vi "BlackBox_filtered.vi"() -> ()   [LabVIEW 2019]
uses:
  <vilib>/Analysis/Matrix/Datatypes/RealMatrix.ctl
  <vilib>/userDefined/High Color/IMAQdx.ctl
  <vilib>/Platform/TimedLoop/XDataNode/timing_clust.ctl
  <vilib>/Platform/TimedLoop/XDataNode/nitl_modes.ctl
  <vilib>/Platform/TimedLoop/XDataNode/wakeup.ctl
  <vilib>/myRIO/Instrument Drivers/Onboard IO/AO/typedefs/AO Reference.ctl
  <vilib>/myRIO/Common/Instrument Driver Framework/Utilities/typedefs/myRIO Generic Hardware Reference.ctl
  <vilib>/myRIO/Common/Instrument Driver Framework/Utilities/typedefs/Hardware Version Enum.ctl
  <vilib>/myRIO/Common/Instrument Driver Framework/Utilities/typedefs/myRIO v1.0 Reference.ctl
  <vilib>/myRIO/Common/Instrument Driver Framework/Utilities/typedefs/Generic FPGA Reference.ctl
  <vilib>/myRIO/Common/Instrument Driver Framework/myRIO v1.0/AO/typedefs/AO Channels List.ctl
  <vilib>/myRIO/Common/Instrument Driver Framework/myRIO v1.0/AO/typedefs/AO Channels Enum.ctl
  <vilib>/myRIO/Common/Instrument Driver Framework/Utilities/typedefs/Analog Scaling Constants List.ctl
  <vilib>/myRIO/Common/Instrument Driver Framework/Utilities/typedefs/Analog Scaling Constants.ctl
  <vilib>/userDefined/High Color/nirio_resource_hc.ctl
  <vilib>/myRIO/Common/Instrument Driver Framework/myRIO v1.0/Encoder/typedefs/Encoder Signal Mode.ctl
  <vilib>/myRIO/Instrument Drivers/Onboard IO/Encoder/typedefs/Encoder Reference.ctl
  <vilib>/myRIO/Common/Instrument Driver Framework/myRIO v1.0/Encoder/typedefs/Encoder Channels Enum.ctl
  <vilib>/myRIO/Common/Instrument Driver Framework/myRIO v1.0/Encoder/typedefs/Encoder Configuration v1.0.ctl
  <vilib>/myRIO/Common/Instrument Driver Framework/Utilities/vis/Is FPGA Ref Available.vi
  <vilib>/myRIO/Common/Instrument Driver Framework/myRIO v1.0/AO/vis/myRIO v1.1 Open AO.vi
  <vilib>/myRIO/Instrument Drivers/Onboard IO/AO/vis/Write.vi
  <vilib>/myRIO/Common/Instrument Driver Framework/myRIO v1.0/Encoder/vis/myRIO v1.1 Open Encoder.vi
  <vilib>/myRIO/Instrument Drivers/Onboard IO/Encoder/vis/Read.vi
  <vilib>/myRIO/Common/Instrument Driver Framework/Utilities/vis/Validate Channels.vi
  <vilib>/myRIO/Common/Instrument Driver Framework/myRIO v1.0/AO/vis/myRIO v1.0 Reserve AO.vi
  <vilib>/myRIO/Common/Instrument Driver Framework/myRIO v1.0/Encoder/vis/myRIO v1.0 Reserve Encoder.vi
  <vilib>/Analysis/baseanly.llb/A x B.vi
  <vilib>/Analysis/baseanly.llb/A x Vector.vi
  <vilib>/myRIO/Common/Instrument Driver Framework/myRIO v1.0/AO/vis/myRIO v1.0 Build MUX Configuration AO.vi
  <vilib>/myRIO/Common/Instrument Driver Framework/myRIO v1.0/Resource Manager/vis/myRIO v1.0 Reserve Channel List.vi
  <vilib>/myRIO/Common/Instrument Driver Framework/myRIO v1.0/Encoder/vis/myRIO v1.0 Build MUX Configuration Encoder.vi
  <vilib>/myRIO/Common/Instrument Driver Framework/myRIO v1.0/Resource Manager/vis/myRIO v1.0 Reserve Channel.vi
  <vilib>/myRIO/Common/Instrument Driver Framework/myRIO v1.0/Resource Manager/vis/myRIO v1.0 Unreserve Channel.vi
  <vilib>/myRIO/Common/Instrument Driver Framework/myRIO v1.0/Resource Manager/vis/myRIO v1.0 Create Configuration List.vi
  <vilib>/myRIO/Common/Instrument Driver Framework/myRIO v1.0/Resource Manager/vis/myRIO v1.0 Build Mutex Name.vi
  <vilib>/Utility/VariantDataType/GetNumericInfo.vi
  <vilib>/Utility/error.llb/Error Cluster From Error Code.vi
  <vilib>/myRIO/Common/Instrument Driver Framework/myRIO v1.0/myRIO v1.1 Open.vi
  <vilib>/myRIO/Common/Instrument Driver Framework/myRIO v1.0/AO/vis/myRIO v1.0 Get Scaling Constants AO.vi
  <vilib>/myRIO/Common/Instrument Driver Framework/Utilities/vis/IO Manager.vi
  <vilib>/myRIO/Common/Instrument Driver Framework/Utilities/vis/Configuration Manager.vi
  <vilib>/myRIO/Common/Instrument Driver Framework/myRIO v1.0/myRIO v1.0 Close.vi
  <vilib>/myRIO/Common/Instrument Driver Framework/myRIO v1.0/AO/vis/myRIO v1.0 Write AO.vi
  <vilib>/Utility/file.llb/Write Delimited Spreadsheet (DBL).vi
  <vilib>/myRIO/Common/Instrument Driver Framework/myRIO v1.0/Resource Manager/vis/myRIO v1.0 Configure IO.vi
  <vilib>/myRIO/Common/Instrument Driver Framework/myRIO v1.0/Encoder/vis/myRIO v1.0 Configure Encoder.vi
  <vilib>/myRIO/Common/Instrument Driver Framework/myRIO v1.0/Encoder/vis/myRIO v1.0 Read Encoder.vi
  <vilib>/platform/TimedLoop/XDataNode/XDataNode.xnode
  <vilib>/myRIO/Express VI/Onboard IO/AO/AO Express VI.xnode
  <vilib>/myRIO/Instrument Drivers/Onboard IO/AO/vis/myRIO AO Open.xnode
  <vilib>/myRIO/Express VI/Onboard IO/Encoder/Encoder Express VI.xnode
  <vilib>/myRIO/Instrument Drivers/Onboard IO/Encoder/vis/myRIO Encoder Open.xnode
  <vilib>/myRIO/Common/Instrument Driver Framework/myRIO v1.0/Encoder/typedefs/Encoder Count Direction Enum.ctl
  <vilib>/Platform/TimedLoop/XDataNode/XDNodeRunTimeDep.lvlib
  <vilib>/myRIO/Instrument Drivers/Onboard IO/AO/AO.lvlib
  <vilib>/vision/driver/NI_Vision_Acquisition_Software.lvlib
  <vilib>/myRIO/Instrument Drivers/Onboard IO/Encoder/Encoder.lvlib
  <vilib>/vision/NI_Vision_Development_Module.lvlib
  <vilib>/Analysis/Matrix/NI_Matrix.lvlib
panel:
  out "deltaT":u32
  out "scaled_obs_y":dbl[](array[numeric])
  out "scaled_obs_x":dbl[](array[numeric])
  out "done":bool
  out "target_y":dbl
  out "target_x":dbl
  in  "start_test":bool
  out "observation":dbl[](array[numeric])
  out "scaled_obs":dbl[](array[numeric])
  in  "record_name":string
  out "record":T1
  out "step_recorded":dbl
  in  "stop_recording":bool
  in  "start_recording":bool
  out "recording":bool
  out "record_t":dbl[](array[numeric])
  out "target_a_y":dbl(knob) scale=-45.0..45.0
  out "target_a_x":dbl(knob) scale=-45.0..45.0
  out "y_angle":dbl(knob) scale=-45.0..45.0
  out "x_angle":dbl(knob) scale=-45.0..45.0
  out "y_error":dbl
  out "x_error":dbl
  out "y":dbl
  out "x":dbl
  out "camera":T2(plugin-control)
  in  "threshold":cluster{"Lower value":sgl, "Upper value":sgl}={"Lower value"=60.0, "Upper value"=255.0} {"Upper value" format="%.2f"; "Lower value" format="%.2f"}
  out "threshold":T2(plugin-control)
  out "x-y":u32
  out "y_input":dbl
  out "y_angle_error":dbl
  out "x_angle_error":dbl
  in  "stop":bool
  out "x_input":dbl
  in  "reset":bool
  in  "dt":dbl=20.0
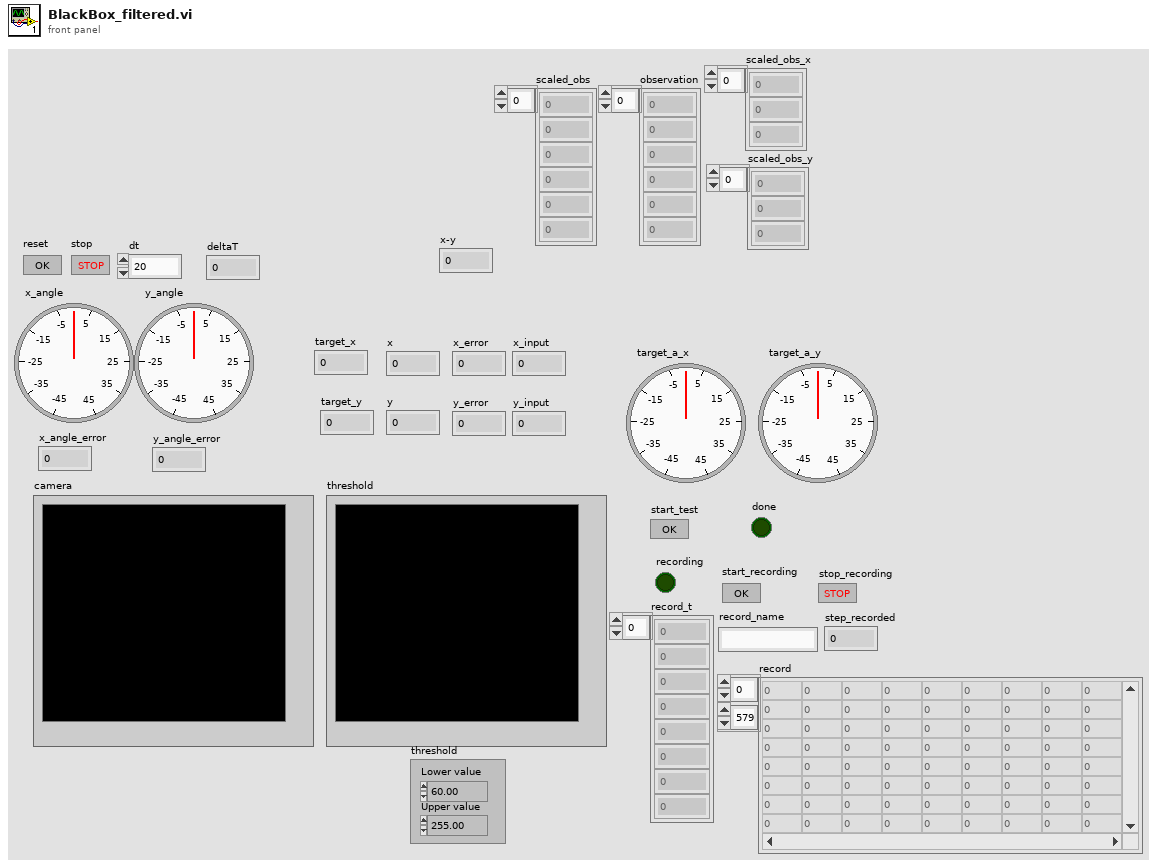
[diagram p1: front panel]
types:
  T1 = typedef "NI_Matrix.lvlib/RealMatrix.ctl" = dbl[][]
  T2 = typedef "IMAQ Image.ctl" = refnum<image>
  T3 = typedef "IMAQdx.ctl" = refnum<k21>
  T4 = typedef "XDNodeRunTimeDep.lvlib/timing_clust.ctl" = cluster{"Expected End [f-1]":u64, "Actual End [f-1]":u64, "Finished Late? [f-1]":bool, "Expected End [i-1]":u64, "Actual End [i-1]":u64, "Finished Late? [i-1]":bool, "Expected Start [i]":u64, "Actual Start [i]":u64, "Expected Start [f]":u64, "Actual Start [f]":u64, "Source Name":string, "Structure Name":string, "Period":i64, "Deadline":i64, "Offset":i64, "Start":i64, "Priority":i32, "Timeout":i32, "Mode":T5, "Wakeup Reason":T6, "Error":errorcluster, "Source Type":string, "Secondary Source Type":string, "Global End Time":u64, "Global Start Time":u64, "Frame Duration":u64, "Iteration Duration":u64, "Assigned CPU":i32, "I/O Scan Engine Mode":u32}
  T5 = typedef "XDNodeRunTimeDep.lvlib/nitl_modes.ctl" = enum32{"No Change", "Process missed periods, maintain original phase", "Discard missed periods, maintain original phase", "Process missed periods, ignore original phase", "Discard missed periods, ignore original phase"}
  T6 = typedef "XDNodeRunTimeDep.lvlib/wakeup.ctl" = enum32{"Normal", "Aborted", "Asynchronous wakeup", "Timing source error", "Timed loop error", "Timeout"}
  T7 = typedef "Encoder.lvlib/Encoder Reference.ctl" = cluster{"myRIO Reference":T8, "Encoder Channels Enum":T12}
  T8 = typedef "myRIO Generic Hardware Reference.ctl" = cluster{"myRIO Model":T9, "myRIO Hardware Reference":T10}
  T9 = typedef "Hardware Version Enum.ctl" = enum16{"Unknown", "myRIO-1900", "myRIO-1950", "roboRIO", "NI ELVIS RIO CM", "ELVIS III"}
  T10 = typedef "myRIO v1.0 Reference.ctl" = cluster{"Generic FPGA Reference":T11, "Allow multiple opens":bool}
  T11 = typedef "Generic FPGA Reference.ctl" = refnum<k20>
  T12 = typedef "Encoder Channels Enum.ctl" = enum16{"Not Connected", "C/ENC0", "C/ENC1", "A/ENC", "A/ENC0", "A/ENC1", "A/ENC2", "A/ENC3", "A/ENC4", "A/ENC5", "A/ENC6", "A/ENC7", "A/ENC8", "A/ENC9", "B/ENC", "B/ENC0", "B/ENC1", "B/ENC2", "B/ENC3", "B/ENC4", "B/ENC5", "B/ENC6", "B/ENC7", "B/ENC8", "B/ENC9", "DIO/ENC0", "DIO/ENC1", "DIO/ENC2", "DIO/ENC3", "DIO/ENC4"}
  T13 = typedef "Encoder Signal Mode.ctl" = enum16{"Quadrature phase signal", "Step and direction signal"}
  T14 = typedef "nirio_resource_hc.ctl" = tag
  T15 = typedef "AO.lvlib/AO Reference.ctl" = cluster{"myRIO Reference":T8, "AO Channel List":T16, "AO Scaling Constant List":T18}
  T16 = typedef "AO Channels List.ctl" = T17[]
  T17 = typedef "AO Channels Enum.ctl" = enum16{"Not Connected", "AudioOut/Left", "AudioOut/Right", "C/AO0", "C/AO1", "A/AO0", "A/AO1", "B/AO0", "B/AO1"}
  T18 = typedef "Analog Scaling Constants List.ctl" = T19[]
  T19 = typedef "Analog Scaling Constants.ctl" = cluster{"LSB Weight (Volts)":dbl, "Offset (Volts)":dbl, "Signed?":bool}
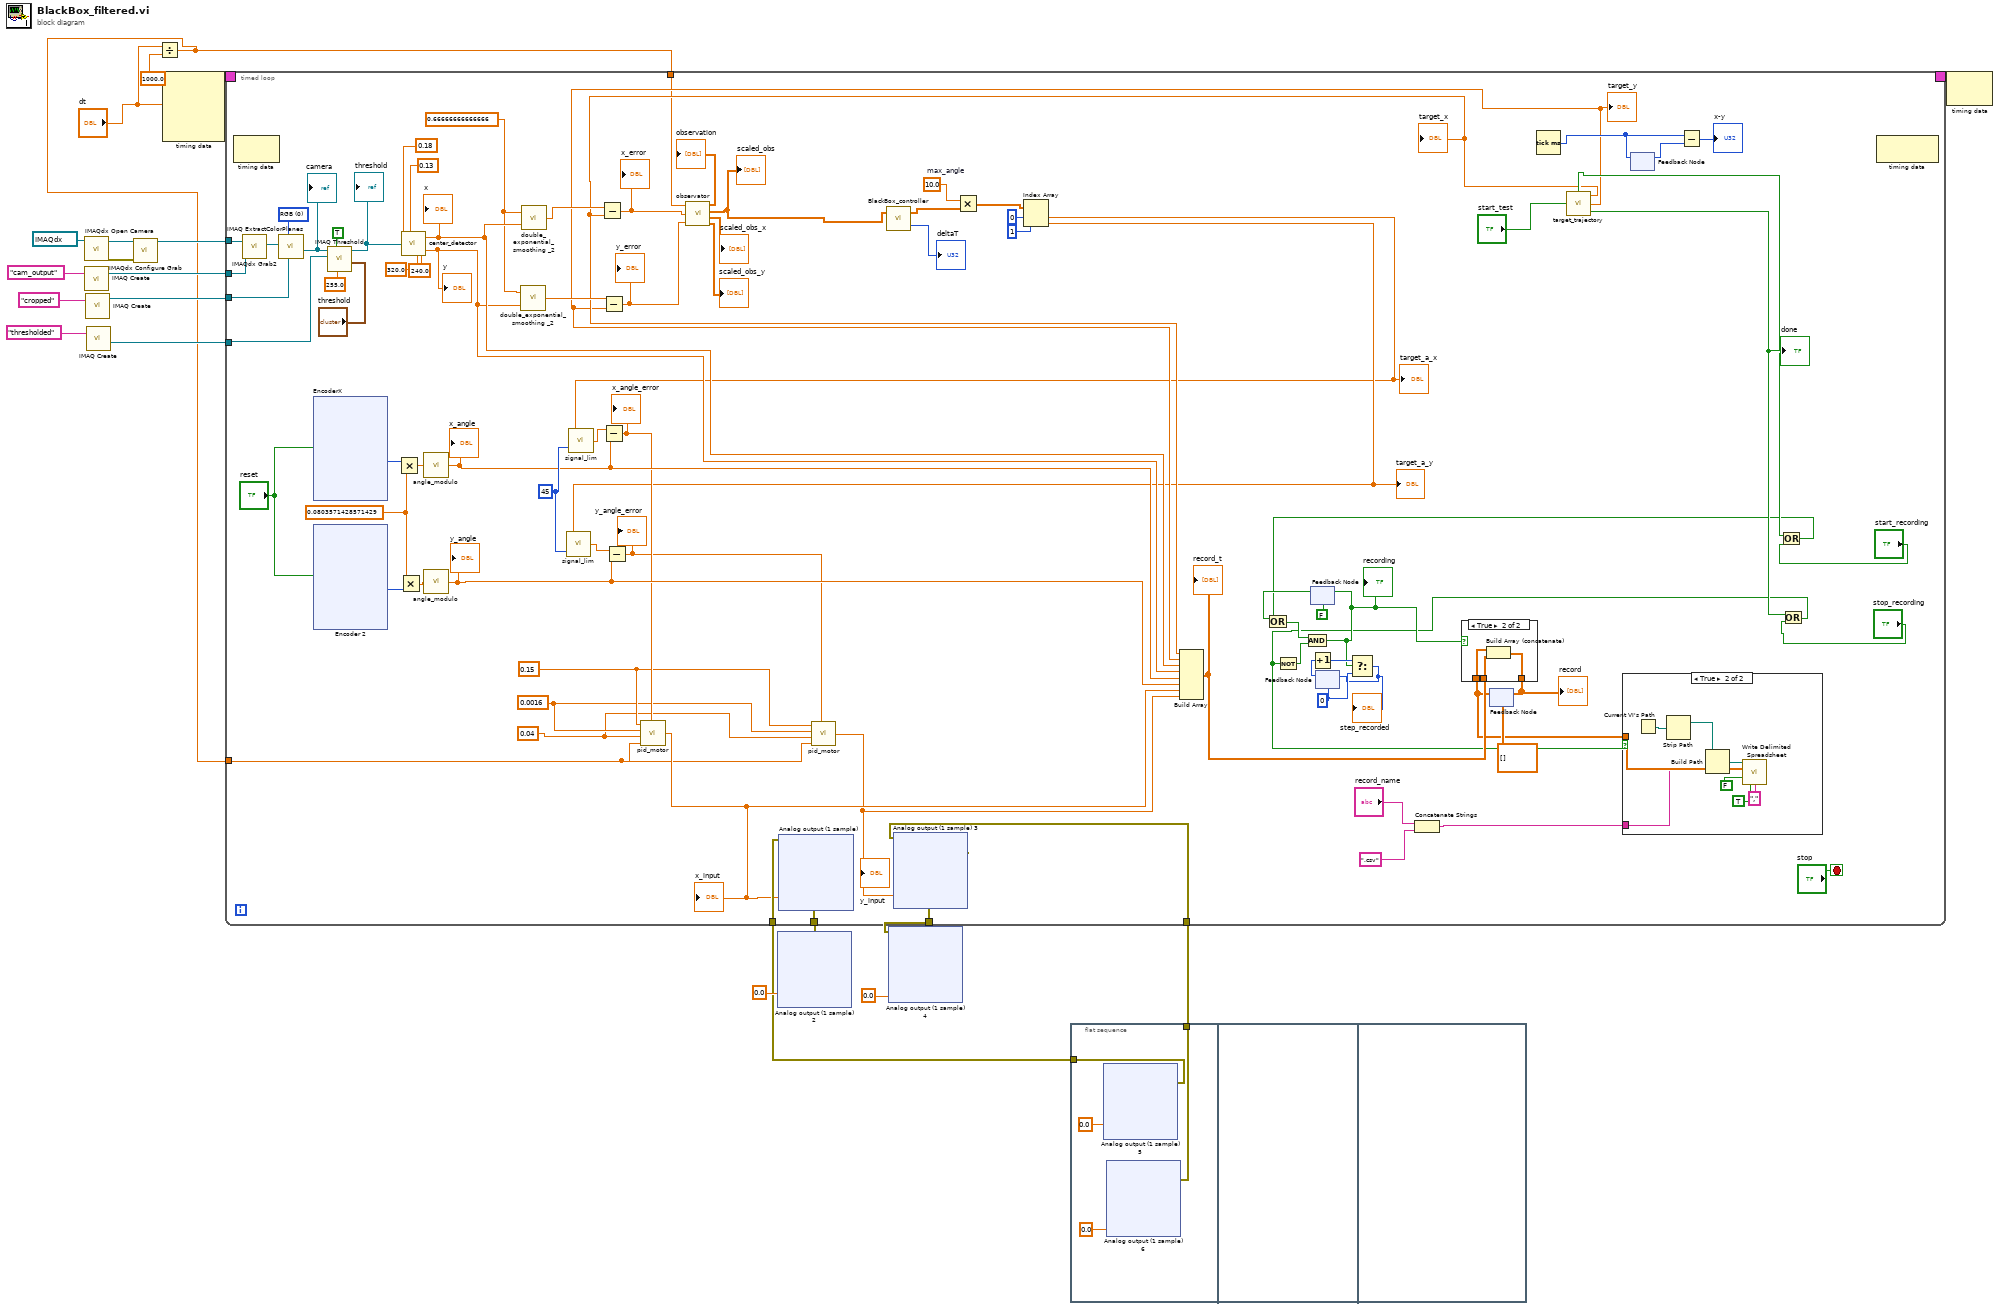
[diagram p0: block diagram]
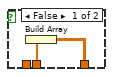
[diagram p3: hidden frame]
diagram:
  n1 = call <vilib>:"IMAQdx Open Camera.vi"("Session In"=T3 "cam2") -> ("error out"=w13:errorcluster, "Session Out"=w14:T3)  [unwired: 9 in]
  n2 = call "IMAQ Create"("Image Name"="cam_output") -> ("New Image"=w15:T2)  [unwired: 4 in, 1 out]
  n3 = call "IMAQ Create"("Image Name"="cropped") -> ("New Image"=w6:T2)  [unwired: 4 in, 1 out]
  n4 = call "IMAQ Create"("Image Name"="thresholded") -> ("New Image"=w4:T2)  [unwired: 4 in, 1 out]
  n5 = call <vilib>:"IMAQdx Configure Grab.vi"("error in"=w13, "Session In"=w14) -> ("Session Out"=w16:T3)  [unwired: 8 in, 1 out]
  n6 = Divide(x="dt", y=1000.0) -> (x/y=w1:dbl)
  n7 = node-c288("dt") -> (w21:T4)  [unwired: 3 in]
  n8 = timed-loop {
    timing: w21 -> [_]
    timing-out: [_] -> w20
    tunnel: w16 -> [w108]
    tunnel: w15 -> [w107]
    tunnel: w1 -> [w49]
    tunnel: [w96] -> w11
    tunnel: [w92] -> w10
    tunnel: w9 -> [w91]
    tunnel: w8 -> [w90]
    tunnel: w6 -> [w65]
    tunnel: w4 -> [w59]
    tunnel: w1 -> [w37]
    stop <- "stop" stop-if-true
    w23 = 10.0  # max_angle
    w54 = 0.66666666666666
    w46 = 0.04 ("ki")
    w47 = 0.0016 ("kd")
    w48 = 0.15 ("kp")
    w68 = u16 0 items=["RGB", "HSL", "HSV", "HSI"] ("Color Mode")
    w78 = 0
    w97 = 45
    w105 = 0.0803571428571429
    n9 = node-c288() -> ()  [unwired: 1 in, 1 out]
    n10 = call <vilib>:"IMAQdx Grab2.vi"("Image In"=w107, "Session In"=w108) -> ("Image Out"=w67:T2)  [unwired: 6 in, 3 out]
    n11 = call "IMAQ ExtractColorPlanes"("Blue or Luma or Val or Inten Plane"=w65, "Color Mode"=w68, "Image Src"=w67) -> ("Blue or Luma or Val or Inten Plane out"=w66:T2)  [unwired: 5 in, 3 out]
    "camera" <- w66
    n12 = xnode "EncoderX"("Reset Counter"="reset") -> ("Counter Value"=w106:i32)  [unwired: 1 in, 3 out]
    n13 = xnode "Encoder 2"("Reset Counter"="reset") -> ("Counter Value"=w104:i32)  [unwired: 1 in, 3 out]
    n14 = call "IMAQ Threshold"("Replace Value"=sgl 255.0, "Keep/Replace Value (Replace)"=TRUE, "Range"="threshold", "Image Dst"=w59, "Image Src"=w66) -> ("Image Dst Out"=w62:T2)  [unwired: 5 in, 1 out]
    "threshold" <- w62
    n15 = Multiply(x=w106, y=w105) -> (x*y=w101:dbl)
    n16 = Multiply(x=w105, y=w104) -> (x*y=w100:dbl)
    n17 = call "center_detector.vi"("px_x"=320.0, "px_y"=240.0, "Image"=w62, "m_x"=0.18, "m_y"=0.13) -> ("x"=w57:dbl, "y"=w55:dbl)
    "x" <- w57
    "y" <- w55
    n18 = call "angle_modulo.vi"("alpha"=w101) -> ("alpha_prime"=w86:dbl)
    "x_angle" <- w86
    n19 = call "angle_modulo.vi"("alpha"=w100) -> ("alpha_prime"=w85:dbl)
    "y_angle" <- w85
    n20 = call "double_exponential_smoothing _2.vi"("x"=w55, "alpha"=w54) -> ("dema"=w56:dbl)
    n21 = call "double_exponential_smoothing _2.vi"("x"=w57, "alpha"=w54) -> ("dema"=w58:dbl)
    n22 = feedback #1(FALSE) -> (w84:bool)
    n23 = feedback #2(w78) -> (w80:i32)
    n24 = Increment(x=w80) -> (x+1=w79:i32)
    n25 = Concatenate Strings("record_name", ".csv") -> (w69:string)
    n26 = feedback #3(T1 [] ("Real Matrix")) -> (w72:T1)
    n27 = Tick Count (ms)() -> (millisecond timer value=w95:u32)
    n28 = call "target_trajectory.vi"("start_test"="start_test") -> ("start"=w42:bool, "target_x"=w39:dbl, "target_y"=w38:dbl, "done"=w43:bool)
    "target_x" <- w39
    "target_y" <- w38
    "done" <- w43
    n29 = Subtract(x=w58, y=w39) -> (x-y=w36:dbl)
    "x_error" <- w36
    n30 = Subtract(x=w56, y=w38) -> (x-y=w35:dbl)
    "y_error" <- w35
    n31 = call "observator.vi"("d_t"=w37, "e_x"=w36, "e_y"=w35) -> ("observation"=→"observation":dbl[], "scaled_obs"=w30:dbl[], "scaled_obs_x"=→"scaled_obs_x":dbl[], "scaled_obs_y"=→"scaled_obs_y":dbl[])
    "scaled_obs" <- w30
    n32 = call "BlackBox_controller.vi"("Normalized observation"=w30) -> ("deltaT"=→"deltaT":u32, "output"=w24:dbl[])  [unwired: 1 in]
    n33 = Multiply(x=w23, y=w24) -> (x*y=w22:dbl[])
    n34 = Index Array(array=w22, index #1=0 ("index"), index #2=1 ("index")) -> (element #1=w25:dbl, element #2=w26:dbl)
    "target_a_x" <- w25
    "target_a_y" <- w26
    n35 = call "signal_lim.vi"("lim"=w97, "x"=w26) -> ("y"=w98:dbl)
    n36 = call "signal_lim.vi"("lim"=w97, "x"=w25) -> ("y"=w99:dbl)
    n37 = Subtract(x=w99, y=w86) -> (x-y=w53:dbl)
    "x_angle_error" <- w53
    n38 = Subtract(x=w98, y=w85) -> (x-y=w51:dbl)
    "y_angle_error" <- w51
    n39 = call "pid_motor.vi"("kp"=w48, "kd"=w47, "ki"=w46, "dt"=w49, "err"=w53) -> ("u"=w52:dbl)
    "x_input" <- w52
    n40 = xnode "Analog output (1 sample)"("C/AO0 (AO0)"=w52, "error in (no error)"=w91) -> ("error out"=w96:errorcluster)
    n41 = call "pid_motor.vi"("kp"=w48, "kd"=w47, "ki"=w46, "dt"=w49, "err"=w51) -> ("u"=w50:dbl)
    "y_input" <- w50
    n42 = xnode "Analog output (1 sample) 3"("C/AO1 (AO1)"=w50, "error in (no error)"=w90) -> ("error out"=w92:errorcluster)
    n43 = Build Array(w39, w38, w57, w55, w86, w85, w52, w50) -> (w75:dbl[])
    "record_t" <- w75
    n44 = feedback-in #4(w95) -> ()
    n45 = feedback #4() -> (w94:u32)  [unwired: 1 in]
    n46 = Subtract(x=w95, y=w94) -> (x-y=→"x-y":u32)
    n47 = Or(x=w42, y="start_recording") -> (x .or. y?=w41:bool)
    n48 = Or(x=w84, y=w41) -> (x .or. y?=w83:bool)
    n49 = Or(x=w43, y="stop_recording") -> (x .or. y?=w31:bool)
    n50 = Not(x=w31) -> (.not. x?=w82:bool)
    n51 = And(x=w83, y=w82) -> (x .and. y?=w76:bool)
    "recording" <- w76
    n52 = feedback-in #1(w76) -> ()
    n53 = Select(t=w79, s=w76, f=w78) -> (s? t:f=w77:i32)
    "step_recorded" <- w77
    n54 = feedback-in #2(w77) -> ()
    n55 = case shown="True" w76 {
      tunnel: w72 -> [_ w121]
      tunnel: [w117 w120] -> w73
      tunnel: w75 -> [w118 w119]
      frame False {
        n56 = Build Array(w118) -> (w117:T1)
      }
      frame True {
        n57 = Build Array (concatenate)(w121, w119) -> (w120:T1)
      }
    }
    "record" <- w73
    n58 = feedback-in #3(w73) -> ()
    n59 = case shown="True" w31 {
      tunnel: w72 -> [_ w116]
      tunnel: w69 -> [_ w114]
      frame False {
      }
      frame True {
        n60 = Current VI's Path() -> (path=w112:path)
        n61 = Strip Path(path=w112) -> (stripped path=w111:path)  [unwired: 1 out]
        n62 = Build Path(base path=w111, name or relative path=w114) -> (appended path=w113:path)
        n63 = call-poly <vilib>:"Write Delimited Spreadsheet.vi"("file path (dialog if empty)"=w113, "2D data"=w116, "append to file? (new file:F)"=FALSE, "transpose? (no:F)"=TRUE, "delimiter (\\t)"="," ("delimiter (\\t)")) -> ()  [unwired: 9 in, 2 out]
      }
    }
    n64 = node-c288() -> ()  [unwired: 1 in, 1 out]
  }
  n65 = xnode "Analog output (1 sample) 2"("C/AO0 (AO0)"=0.0, "error in (no error)"=w11) -> ()  [unwired: 1 out]
  n66 = xnode "Analog output (1 sample) 4"("C/AO1 (AO1)"=0.0, "error in (no error)"=w10) -> ()  [unwired: 1 out]
  n67 = flat-sequence {
    tunnel: [w291] -> w9
    tunnel: [w290] -> w8
    frame #0 {
      n68 = xnode "Analog output (1 sample) 5"("C/AO0 (AO0)"=0.0) -> ("error out"=w291:errorcluster)  [unwired: 1 in]
      n69 = xnode "Analog output (1 sample) 6"("C/AO1 (AO1)"=0.0) -> ("error out"=w290:errorcluster)  [unwired: 1 in]
    }
    frame #1 {
    }
    frame #2 {
    }
  }
  n70 = node-c288(w20) -> ()  [unwired: 1 out]
